vi "Tree Create.vi"(8 "error in (no error)":errorcluster, 10 "Symbols":picture[](array[picture]), 11 "TREE in":refnum<class "MyTreeAPI.lvclass">) -> (0 "error out":errorcluster, 3 "TREE out":refnum<class "MyTreeAPI.lvclass">)   [LabVIEW 2015, in "MyTreeAPI.lvclass"]
uses:
  MyTreeAPI.lvclass
  MyTreeAPI.lvclass/MyTreeAPI.ctl
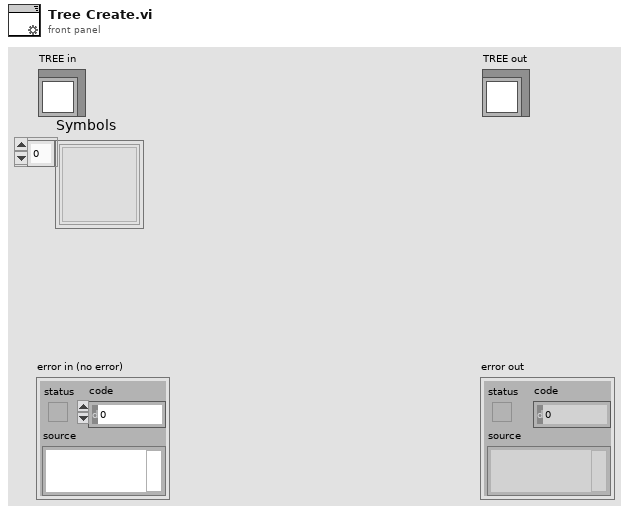
[diagram p1: front panel]
types:
  T1 = typedef "imagedata.ctl" = cluster{"image type":i32, "image depth":i32, "image":u8[], "mask":u8[], "colors":u32[], "Rectangle":cluster{"left":i16, "top":i16, "right":i16, "bottom":i16}}
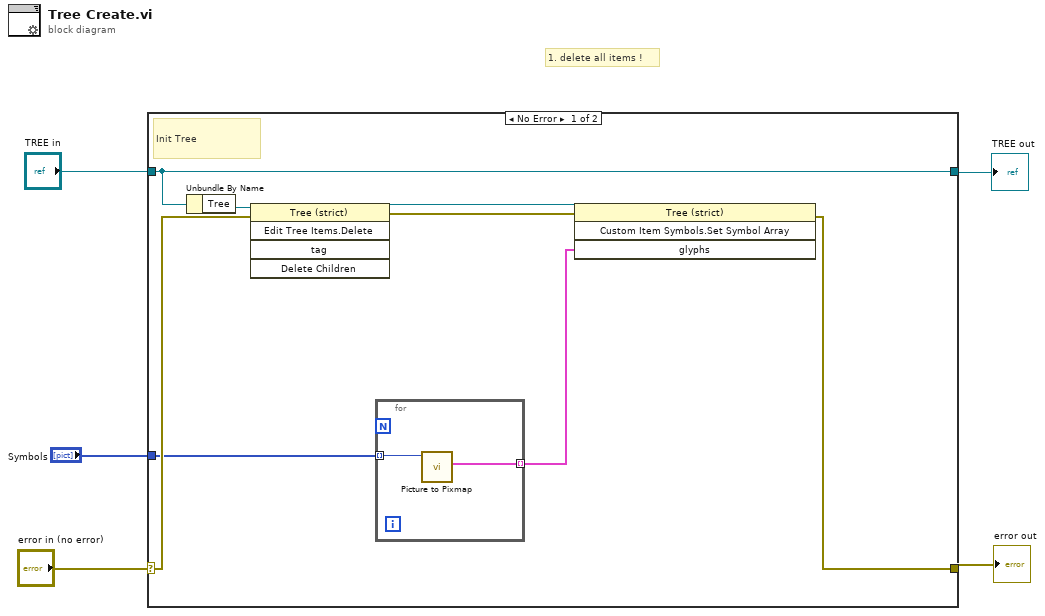
[diagram p0: block diagram]
diagram:
  # "1. delete all items !"
  n1 = case shown="No Error" "error in (no error)" {
    selector: "error in (no error)" -> [w9 w17]
    tunnel: [w7 w17] -> w4
    tunnel: [w6 w16] -> w2
    tunnel: "TREE in" -> [w6 w16]
    tunnel: "Symbols" -> [w8 _]
    frame No Error {
      # "Init Tree"
      n2 = Unbundle By Name(w6) -> ("Tree"=w10:refnum<vi>)
      n3 = invoke class="Tree (strict)" method="Edit Tree Items.Delete"(reference=w10, error in=w9) -> (reference out=w13:refnum<vi>, error out=w12:errorcluster)  [unwired: 3 in, 3 out]
      n4 = for {
        tunnel: w8 -> [w15] mode=indexing
        tunnel: [w14] -> w11 mode=indexing
        n5 = call <vilib>:"Picture to Pixmap.vi"("picture"=w15) -> ("image data"=w14:T1)  [unwired: 9 in, 1 out]
      }
      n6 = invoke class="Tree (strict)" method="Custom Item Symbols.Set Symbol Array"(reference=w13, error in=w12, "glyphs"=w11) -> (error out=w7:errorcluster)  [unwired: 1 in, 3 out]
    }
    frame Error {
    }
  }
  "error out" <- w4
  "TREE out" <- w2
